vi "Testing Notification Abort.vi"() -> ()   [LabVIEW 2021]
panel:
  out "error out 2":errorcluster
  out "error out":errorcluster
  in  "stop":bool
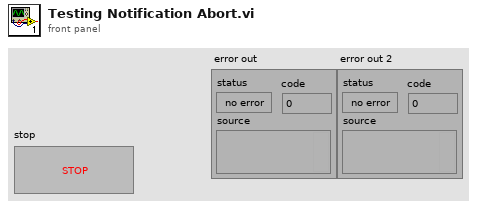
[diagram p1: front panel]
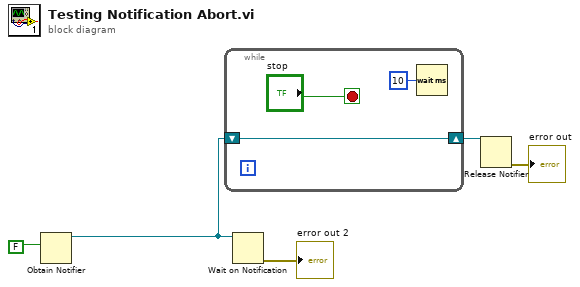
[diagram p0: block diagram]
diagram:
  n1 = Obtain Notifier(notification data type=FALSE) -> (notifier out=w5:refnum<notifier>)  [unwired: 3 in, 2 out]
  n2 = while {
    shift-right: [w6] -> w3
    shift-left: w5 -> [w6]
    stop <- "stop" stop-if-true
    n3 = Wait (ms)(milliseconds to wait=u32 10) -> ()  [unwired: 1 out]
  }
  n4 = Wait on Notification(notifier=w5) -> (error out=→"error out 2":errorcluster)  [unwired: 3 in, 3 out]
  n5 = Release Notifier(notifier=w3) -> (error out=→"error out":errorcluster)  [unwired: 2 in, 2 out]
